vi "Node Config.vi"(8 "error in (no error)":errorcluster, 11 "App in":refnum<class "App.lvclass">) -> (0 "error out":errorcluster, 2 "Node Config":refnum<class "Node Config.lvclass">, 3 "App out":refnum<class "App.lvclass">)   [LabVIEW 2020, in "Volatus.lvlib" / "App.lvclass"]
uses:
  App.lvclass
  App.lvclass/App.ctl
  lv-vecto/Vecto/Node Config/Node Config.lvclass
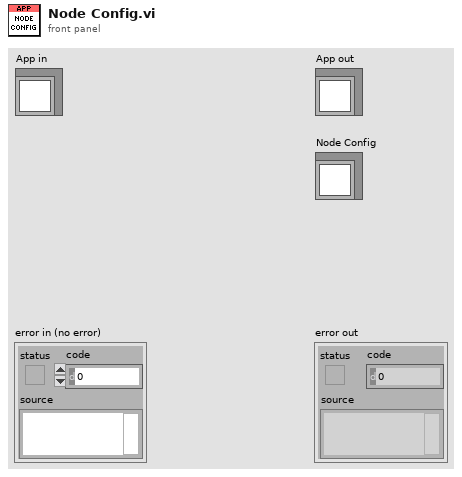
[diagram p1: front panel]
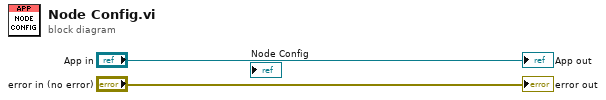
[diagram p0: block diagram]
diagram:
  "error out" <- "error in (no error)"
  "App out" <- "App in"
